vi "Extra_error_Estimates.vi"() -> (5 "Plug in titles":string[](array[string]), 7 "Plug in values":string[](array[string]))   [LabVIEW 2010]
uses:
  Globals/Plug_in_data_global.vi
  Globals/Meas_global.vi
panel:
  in  "Array":u16[][](array[ring])
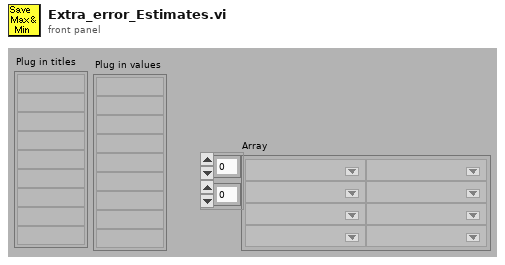
[diagram p1: front panel]
types:
  T1 = typedef "Analysis_info_cluster.ctl" = cluster{"Colour":u32, "Inst type":T2, "Inst name":string, "Symbol":string, "Code name":string, "Extra Info":string, "Inst Array":T3, "Index":i32, "Voltage Index":i32, "Extra Titles":string[], "Extra Values":string[]}
  T2 = typedef "Inst_type.ctl" = enum16{"Propeller anemometer", "Raw voltage", "Pressure Transducer", "Pitot-static tube", "Preston tube", "Hot wire", "Cross wire 1", "Cross wire 2", "Generic Linear", "Generic Polynomial", "Generic BackPoly", "Fast FID", "Thermocouple", "Cold wire", "Pulsed Wire", "LDA Vel", "LDA Tran time", "LDA Arr time"}
  T3 = typedef "Instrument_Array.ctl" = enum16{"PWA", "LDA", "Analogue"}
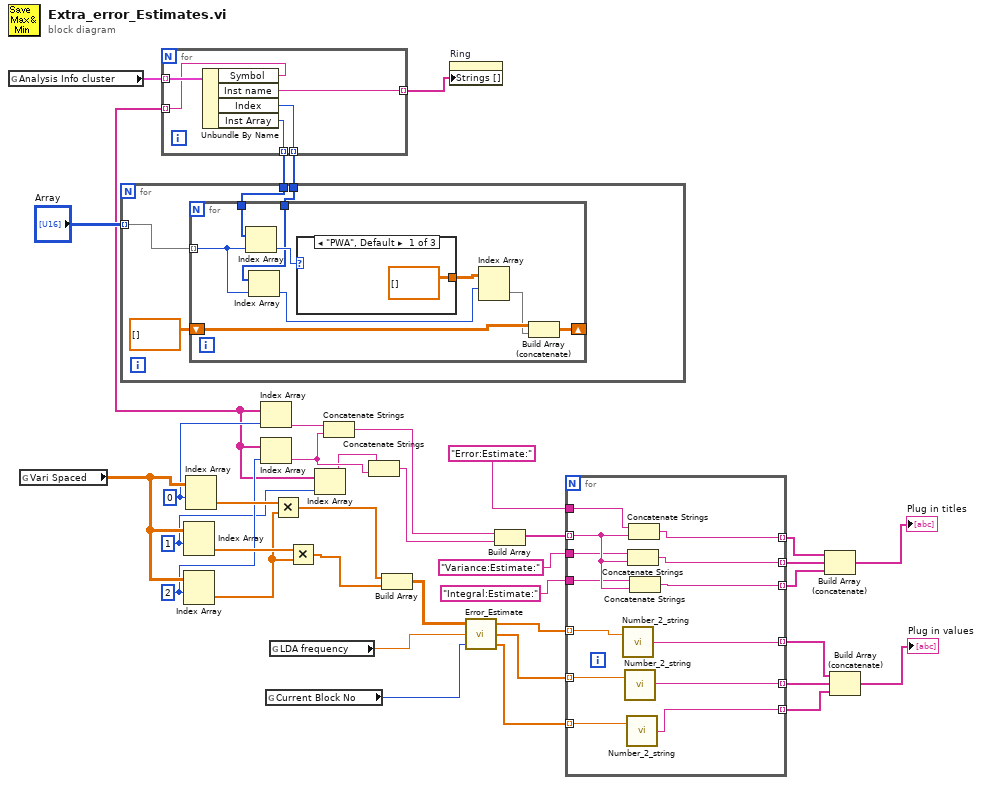
[diagram p0: block diagram]
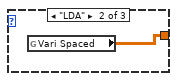
[diagram p2: hidden frame]
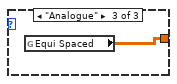
[diagram p3: hidden frame]
diagram:
  w21 = 2 ("index (row)")
  w20 = 1 ("index (row)")
  w22 = 0 ("index (row)")
  n1 = global read "Meas_global.vi" "Analysis Info cluster"() -> (w33:T1[])
  n2 = global read "Plug_in_data_global.vi" "Vari Spaced"() -> (w28:dbl[][])
  n3 = for {
    tunnel: w33 -> [w43] mode=indexing
    tunnel: [w42] -> w32 mode=indexing
    tunnel: [w41] -> w30 mode=indexing
    tunnel: [w40] -> w29 mode=indexing
    tunnel: [w39] -> w19 mode=indexing
    n4 = Unbundle By Name(w43) -> ("Symbol"=w39:string, "Inst name"=w42:string, "Index"=w40:i32, "Inst Array"=w41:T3)
  }
  n5 = for {
    tunnel: "Array" -> [w46] mode=indexing
    tunnel: w30 -> [w47]
    tunnel: w29 -> [w45]
    n6 = for {
      tunnel: w47 -> [w55]
      tunnel: w46 -> [w53] mode=indexing
      tunnel: w45 -> [w52]
      shift-right: [w48] -> _
      shift-left: dbl[][] [] -> [w50]
      n7 = Index Array(array=w55, index=w53) -> (element=w56:T3)
      n8 = Index Array(array=w52, index=w53) -> (element=w51:i32)
      n9 = case shown="\"PWA\", Default" w56 {
        tunnel: [dbl[][] [] ("Equi Spaced") w58 w59] -> w54
        frame "PWA", Default {
        }
        frame "LDA" {
          n10 = global read "Plug_in_data_global.vi" "Vari Spaced"() -> (w58:dbl[][])
        }
        frame "Analogue" {
          n11 = global read "Plug_in_data_global.vi" "Equi Spaced"() -> (w59:dbl[][])
        }
      }
      n12 = Index Array(array=w54, index (row)=w51) -> (element=w49:dbl[])  [unwired: 1 in]
      n13 = Build Array (concatenate)(w50, w49) -> (w48:dbl[][])
    }
  }
  n14 = Index Array(array=w28, index (row)=w20) -> (element=w26:dbl[])  [unwired: 1 in]
  n15 = Index Array(array=w28, index (row)=w21) -> (element=w25:dbl[])  [unwired: 1 in]
  n16 = Index Array(array=w28, index (row)=w22) -> (element=w27:dbl[])  [unwired: 1 in]
  n17 = Index Array(array=w19, index=w22) -> (element=w18:string)
  n18 = Index Array(array=w19, index=w21) -> (element=w15:string)
  n19 = global read "Meas_global.vi" "Current Block No"() -> (w37:i32)
  n20 = global read "Meas_global.vi" "LDA frequency"() -> (w38:dbl)
  n21 = Multiply(x=w27, y=w25) -> (x*y=w24:dbl[])
  n22 = Multiply(x=w26, y=w25) -> (x*y=w23:dbl[])
  n23 = Index Array(array=w19, index=w20) -> (element=w14:string)
  n24 = Concatenate Strings(w18, w15) -> (w17:string)
  n25 = Concatenate Strings(w14, w15) -> (w13:string)
  n26 = Build Array(w24, w23) -> (w36:dbl[][])
  n27 = property on="Ring" class="Ring (strict)"("Strings []"=w32) -> ()  [unwired: 2 in, 2 out]
  n28 = call "Error_Estimate.vi"("Block No"=w37, "Sampling Frequency (Hz)"=w38, "Data In"=w36) -> ("Integral to 25%"=w5:dbl[], "Variance"=w6:dbl[], "Error Estimates"=w34:dbl[])
  n29 = Build Array(w17, w13) -> (w16:string[])
  n30 = for {
    tunnel: "Error:Estimate:" -> [w71]
    tunnel: [w70] -> w10 mode=indexing
    tunnel: w34 -> [w72] mode=indexing
    tunnel: [w69] -> w4 mode=indexing
    tunnel: w16 -> [w68] mode=indexing
    tunnel: "Variance:Estimate:" -> [w67]
    tunnel: "Integral:Estimate:" -> [w66]
    tunnel: [w65] -> w9 mode=indexing
    tunnel: [w64] -> w8 mode=indexing
    tunnel: w6 -> [w63] mode=indexing
    tunnel: w5 -> [w62] mode=indexing
    tunnel: [w61] -> w3 mode=indexing
    tunnel: [w60] -> w2 mode=indexing
    n31 = call "Number_2_string.vi"("number"=w72) -> ("String"=w69:string)  [unwired: 1 in]
    n32 = call "Number_2_string.vi"("number"=w63) -> ("String"=w61:string)  [unwired: 1 in]
    n33 = call "Number_2_string.vi"("number"=w62) -> ("String"=w60:string)  [unwired: 1 in]
    n34 = Concatenate Strings(w67, w68) -> (w65:string)
    n35 = Concatenate Strings(w71, w68) -> (w70:string)
    n36 = Concatenate Strings(w66, w68) -> (w64:string)
  }
  n37 = Build Array (concatenate)(w10, w9, w8) -> (→"Plug in titles":string[])
  n38 = Build Array (concatenate)(w4, w3, w2) -> (→"Plug in values":string[])
